vi "avg all signals.vi"(7 "error in (no error)":errorcluster, 8 "reset averaging":bool, 10 "processing loop vars":T1 {"CurrInverter"."last updated" format="%<%H:%M\n%d/%m/%Y>T"; "CurrInverter"."set flag" items=["False", "True"]}) -> (0 "error out":errorcluster, 2 "Average scaled ESR sum":dbl[](array[numeric]), 3 "processing loop vars out":T1 {"CurrInverter"."last updated" format="%<%H:%M\n%d/%m/%Y>T"; "CurrInverter"."set flag" items=["False", "True"]})   [LabVIEW 2019, in "Main.lvclass"]
doc: "Developed by Kevin Thompson\nkevin@thompsonengineering.net\n\nCopyright 2020\nThompson Engineering, LLC"
uses:
  Main.lvclass
  DataTypes/Processing loop variables--cluster.ctl
  DataTypes/averaging variables.ctl
  DataTypes/ESR alarm variables.ctl
  Common/DataTypes/Inverter database record v2--cluster.ctl
  Common/DataTypes/inverter info v2--cluster.ctl
  Common/DataTypes/inverter gain range--cluster.ctl
  Common/DataTypes/inverter offset range--cluster.ctl
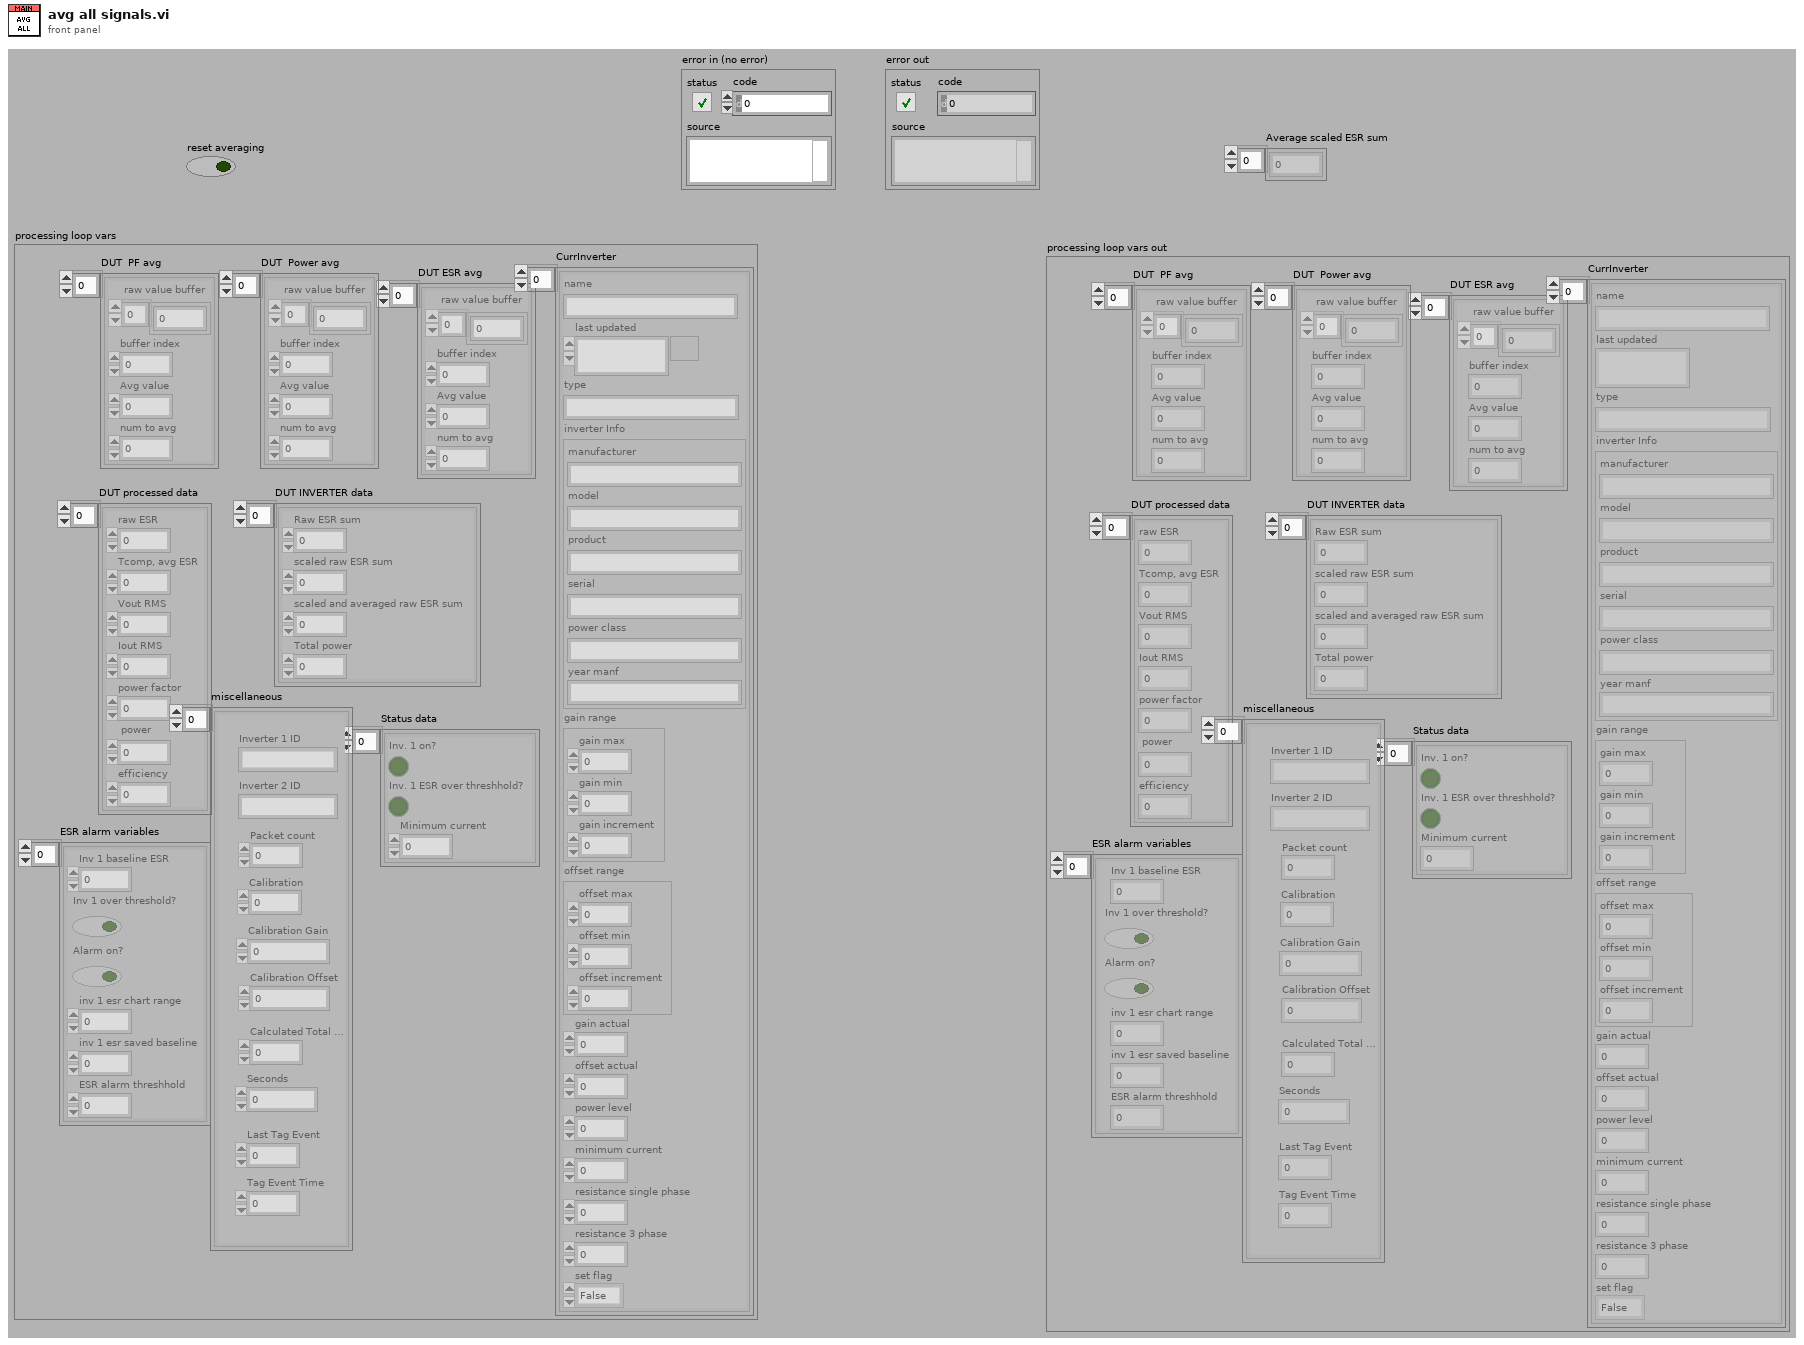
[diagram p1: front panel]
types:
  T1 = typedef "Main.lvclass/Processing loop variables--cluster.ctl" = cluster{"DUT ESR avg":T2[], "DUT  PF avg":T2[], "DUT  Power avg ":T2[], "DUT processed data":cluster{"raw ESR":dbl, "Tcomp, avg ESR":dbl, "Vout RMS":dbl, "Iout RMS":dbl, "power factor":dbl, "power":dbl, "efficiency":dbl}[], "ESR alarm variables":T3[], "Status data":cluster{"Inv. 1 on?":bool, "Inv. 1 ESR over threshhold?":bool, "Minimum current":dbl}[], "CurrInverter":T4[], "miscellaneous":cluster{"Inverter 1 ID":string, "Inverter 2 ID":string, "Packet count":u32, "Calibration":dbl, "Calibration Gain":dbl, "Calibration Offset":dbl, "Calculated Total Power":dbl, "Seconds":dbl, "Last Tag Event":dbl, "Tag Event Time":dbl}[], "DUT INVERTER data":cluster{"Raw ESR sum":dbl, "scaled raw ESR sum":dbl, "scaled and averaged raw ESR sum":dbl, "Total power":dbl}[]}
  T2 = typedef "Main.lvclass/averaging variables.ctl" = cluster{"raw value buffer":dbl[], "buffer index":i32, "Avg value":dbl, "num to avg":i32}
  T3 = typedef "Main.lvclass/ESR alarm variables.ctl" = cluster{"Inv 1 baseline ESR":dbl, "Inv 1 over threshold?":bool, "Alarm on?":bool, "inv 1 esr chart range":dbl, "inv 1 esr saved baseline":dbl, "ESR alarm threshhold":dbl}
  T4 = typedef "Inverter database record v2--cluster.ctl" = cluster{"name":string, "last updated":timestamp, "type":string, "inverter Info":T5, "gain range":T6, "offset range":T7, "gain actual":dbl, "offset actual":dbl, "power level":dbl, "minimum current":dbl, "resistance single phase":dbl, "resistance 3 phase":dbl, "set flag":u16}
  T5 = typedef "inverter info v2--cluster.ctl" = cluster{"manufacturer":string, "model":string, "product":string, "serial":string, "power class":string, "year manf":string}
  T6 = typedef "inverter gain range--cluster.ctl" = cluster{"gain max":dbl, "gain min":dbl, "gain increment":dbl}
  T7 = typedef "inverter offset range--cluster.ctl" = cluster{"offset max":dbl, "offset min":dbl, "offset increment":dbl}
  T8 = cluster{"Raw ESR sum":dbl, "scaled raw ESR sum":dbl, "scaled and averaged raw ESR sum":dbl, "Total power":dbl}[]
  T9 = cluster{"raw ESR":dbl, "Tcomp, avg ESR":dbl, "Vout RMS":dbl, "Iout RMS":dbl, "power factor":dbl, "power":dbl, "efficiency":dbl}[]
  T10 = cluster{"Raw ESR sum":dbl, "scaled raw ESR sum":dbl, "scaled and averaged raw ESR sum":dbl, "Total power":dbl}
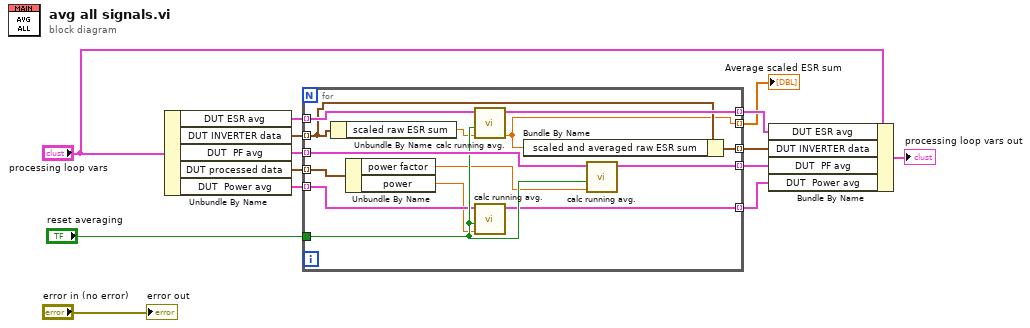
[diagram p0: block diagram]
diagram:
  n1 = Unbundle By Name("processing loop vars") -> ("DUT ESR avg"=w14:T2[], "DUT INVERTER data"=w13:T8, "DUT  PF avg"=w10:T2[], "DUT processed data"=w9:T9, "DUT  Power avg"=w4:T2[])
  n2 = for {
    tunnel: w10 -> [w26] mode=indexing
    tunnel: w9 -> [w25] mode=indexing
    tunnel: "reset averaging" -> [w24]
    tunnel: [w23] -> w5 mode=indexing
    tunnel: w4 -> [w22] mode=indexing
    tunnel: [w21] -> w3 mode=indexing
    tunnel: w14 -> [w28] mode=indexing
    tunnel: [w27] -> w11 mode=indexing
    tunnel: w13 -> [w17] mode=indexing
    tunnel: [w16] -> w2 mode=indexing
    tunnel: [w15] -> w1 mode=indexing
    n3 = Unbundle By Name(w17) -> ("scaled raw ESR sum"=w18:dbl)
    n4 = Unbundle By Name(w25) -> ("power factor"=w20:dbl, "power"=w19:dbl)
    n5 = call "calc running avg..vi"("new val"=w18, "reset?"=w24, "Averaging variables"=w28) -> ("Average val"=w15:dbl, "Averaging variables out"=w27:T2)  [unwired: 7 in]
    n6 = call "calc running avg..vi"("new val"=w19, "reset?"=w24, "Averaging variables"=w22) -> ("Averaging variables out"=w21:T2)  [unwired: 7 in, 1 out]
    n7 = Bundle By Name(cluster=w17, "scaled and averaged raw ESR sum"=w15) -> (w16:T10)
    n8 = call "calc running avg..vi"("new val"=w20, "reset?"=w24, "Averaging variables"=w26) -> ("Averaging variables out"=w23:T2)  [unwired: 7 in, 1 out]
  }
  "Average scaled ESR sum" <- w1
  n9 = Bundle By Name(cluster="processing loop vars", "DUT ESR avg"=w11, "DUT INVERTER data"=w2, "DUT  PF avg"=w5, "DUT  Power avg"=w3) -> (→"processing loop vars out":T1)
  "error out" <- "error in (no error)"
